vi "Registry Set.vi"() -> ()   [LabVIEW 2013]
uses:
  <vilib>/Rock Robotics/WPI/Joystick/WPI_JoystickDeviceEnum.ctl
  <vilib>/Rock Robotics/SystemInterfaces/AI/FPGA_AIChannel.ctl
  <vilib>/Rock Robotics/SystemInterfaces/DIO/FPGA_DIOPWMChannel.ctl
  <vilib>/Rock Robotics/SystemInterfaces/Typedef/FPGA_TypedefAnalogModule.ctl
  <vilib>/Rock Robotics/SystemInterfaces/Typedef/FPGA_TypedefDigitalModule.ctl
  <vilib>/Rock Robotics/SystemInterfaces/DIO/FPGA_DIORelayChannel.ctl
  <vilib>/Rock Robotics/SystemInterfaces/DIO/FPGA_DIOChannel.ctl
  <vilib>/Rock Robotics/WPI/Solenoid/WPI_SolenoidChannel.ctl
  <vilib>/Rock Robotics/SystemInterfaces/Typedef/FPGA_TypedefSolenoidModule.ctl
  <vilib>/Rock Robotics/SystemInterfaces/Typedef/FPGA_TypedefAnalogModuleForGyro.ctl
  <vilib>/Rock Robotics/SystemInterfaces/AI/FPGA_AIGyroChannel.ctl
  <vilib>/Rock Robotics/WPI/MotorControl/WPI_MotorControlOpen Talon.vi
  <vilib>/Rock Robotics/WPI/MotorControl/WPI_MotorControlOpen Jaguar.vi
  <vilib>/Rock Robotics/WPI/Solenoid/WPI_SolenoidOpenSingle.vi
  <vilib>/Rock Robotics/WPI/Counter/WPI_CounterDigitalInputToDigitalSource.vi
  Global Refnums.vi
  <vilib>/Rock Robotics/WPI/Compressor/WPI_CompressorGetSetRefNum.vi
panel:
  out "error out":errorcluster
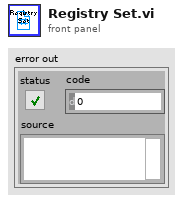
[diagram p1: front panel]
types:
  T1 = typedef "FPGA_AIGyroChannel.ctl" = enum8{"AI 1", "AI 2", "Invalid"}
  T2 = typedef "FPGA_TypedefAnalogModuleForGyro.ctl" = enum16{"Analog Module 1"}
  T3 = typedef "FPGA_DIOChannel.ctl" = enum8{"DIO 1", "DIO 2", "DIO 3", "DIO 4", "DIO 5", "DIO 6", "DIO 7", "DIO 8", "DIO 9", "DIO 10", "DIO 11", "DIO 12", "DIO 13", "DIO 14", "Invalid"}
  T4 = typedef "FPGA_TypedefDigitalModule.ctl" = enum16{"Digital Module 1", "Digital Module 2"}
  T5 = typedef "WPI_SolenoidChannel.ctl" = enum8{"Solenoid 1", "Solenoid 2", "Solenoid 3", "Solenoid 4", "Solenoid 5", "Solenoid 6", "Solenoid 7", "Solenoid 8", "Invalid"}
  T6 = typedef "FPGA_TypedefSolenoidModule.ctl" = enum16{"Solenoid Module 1", "Solenoid Module 2"}
  T7 = typedef "FPGA_DIORelayChannel.ctl" = enum8{"Relay 1", "Relay 2", "Relay 3", "Relay 4", "Relay 5", "Relay 6", "Relay 7", "Relay 8", "Invalid"}
  T8 = typedef "FPGA_DIOPWMChannel.ctl" = enum8{"PWM 1", "PWM 2", "PWM 3", "PWM 4", "PWM 5", "PWM 6", "PWM 7", "PWM 8", "PWM 9", "PWM 10", "Invalid"}
  T9 = typedef "WPI_JoystickDeviceEnum.ctl" = enum16{"USB 1", "USB 2", "USB 3", "USB 4", "Kinect 1", "Kinect 2"}
  T10 = typedef "FPGA_AIChannel.ctl" = enum8{"AI 1", "AI 2", "AI 3", "AI 4", "AI 5", "AI 6", "AI 7", "AI 8", "Invalid"}
  T11 = typedef "FPGA_TypedefAnalogModule.ctl" = enum16{"Analog Module 1", "Analog Module 2"}
  T12 = typedef "WPI_GyroDevRef.ctl" = cluster{"DevStatus":errorcluster, "Analog Module":T11, "Analog Channel":T10, "Offset":dbl, "Gain (VoltsPerDegree/Second)":dbl}
  T13 = typedef "WPI_JoystickDevRef.ctl" = cluster{"Device":T9}
  T14 = typedef "WPI_AnalogChannelDevRef.ctl" = cluster{"DevStatus":errorcluster, "Analog Module":T11, "Analog Channel":T10}
  T15 = typedef "WPI_DigitalInputDevRef.ctl" = cluster{"DevStatus":errorcluster, "DIO Channel":T3, "Digital Module":T4}
  T16 = typedef "WPI_MotorControlDeviceRef.ctl" = cluster{"DeviceStatus":errorcluster, "Type":enum16{"PWM", "CAN"}, "PWM":cluster{"Digital Module":T4, "PWM Channel":T8, "DeadBand":T17}, "CAN":cluster{"Device Number":u8, "Control Mode":T18, "Semaphore":T19, "Max Vout":dbl}, "Invert":bool, "TransformRef":T20, "InvTransformRef":T20}
  T17 = typedef "WPI_PWMDeadband.ctl" = cluster{"Name":string, "maxPositivePwm":i32, "minPositivePwm":i32, "centerPwm":i32, "maxNegativePwm":i32, "minNegativePwm":i32, "angularRange":u16}
  T18 = typedef "WPI_CANJaguar_ControlMode.ctl" = enum8{"Percent VBus", "Current", "Speed", "Position", "Voltage"}
  T19 = typedef "Semaphore RefNum" = refnum<k1>
  T20 = typedef "WPI_PWMTransform_ConPane.ctl" = refnum<vi>
  T21 = typedef "FPGA_CounterEncoderSourceConvertionLVSourceType.ctl" = cluster{"DevStatus":errorcluster, "AnalogTriggerMode?":bool, "DigitalMode":cluster{"Digital Module":T4, "DIO Channel":T22}, "AnalogTriggerMode":cluster{"AnalogTriggerIndex":T23, "OutputType":T24}}
  T22 = typedef "FPGA_DIODigitalSourceChannel.ctl" = enum8{"DIO 1", "DIO 2", "DIO 3", "DIO 4", "DIO 5", "DIO 6", "DIO 7", "DIO 8", "DIO 9", "DIO 10", "DIO 11", "DIO 12", "DIO 13", "DIO 14", "Disabled"}
  T23 = typedef "FPGA_AnalogTriggerIndex.ctl" = enum8{"Trig 0", "Trig 1", "Trig 2", "Trig 3", "Trig 4", "Trig 5", "Trig 6", "Trig 7", "Invalid"}
  T24 = typedef "FPGA_AnalogTriggerOutType.ctl" = enum16{"InWindow", "TriggerState", "Rising", "Falling"}
  T25 = typedef "WPI_EncoderDevRef.ctl" = cluster{"DevStatus":errorcluster, "EncoderIndex":T26, "CounterIndex":T27, "DistancePerCount":dbl, "Decoding Type":T28}
  T26 = typedef "FPGA_EncoderIdx.ctl" = enum8{"Enc 0", "Enc 1", "Enc 2", "Enc 3", "Invalid"}
  T27 = typedef "FPGA_CounterCtrSystemIndex.ctl" = enum8{"Ctr 0", "Ctr 1", "Ctr 2", "Ctr 3", "Ctr 4", "Ctr 5", "Ctr 6", "Ctr 7", "Invalid"}
  T28 = typedef "WPI_EncoderType.ctl" = enum16{"1x", "2x", "4x"}
  T29 = typedef "WPI_CompressorDevRef.ctl" = cluster{"DevStatus":errorcluster, "DigitalInputDevRef":T15, "RelayDevRef":T30}
  T30 = typedef "WPI_RelayDevRef.ctl" = cluster{"DevStatus":errorcluster, "Relay Channel":T7, "Digital Module":T4, "Relay Direction":T31}
  T31 = typedef "WPI_RelayDirection.ctl" = enum16{"Both directions", "Forward only", "Reverse only"}
  T32 = typedef "WPI_SolenoidDevRef.ctl" = cluster{"DevStatus":errorcluster, "Solenoid Module":T6, "Forward Solenoid Channel":T5, "Reverse Solenoid Channel":T5}
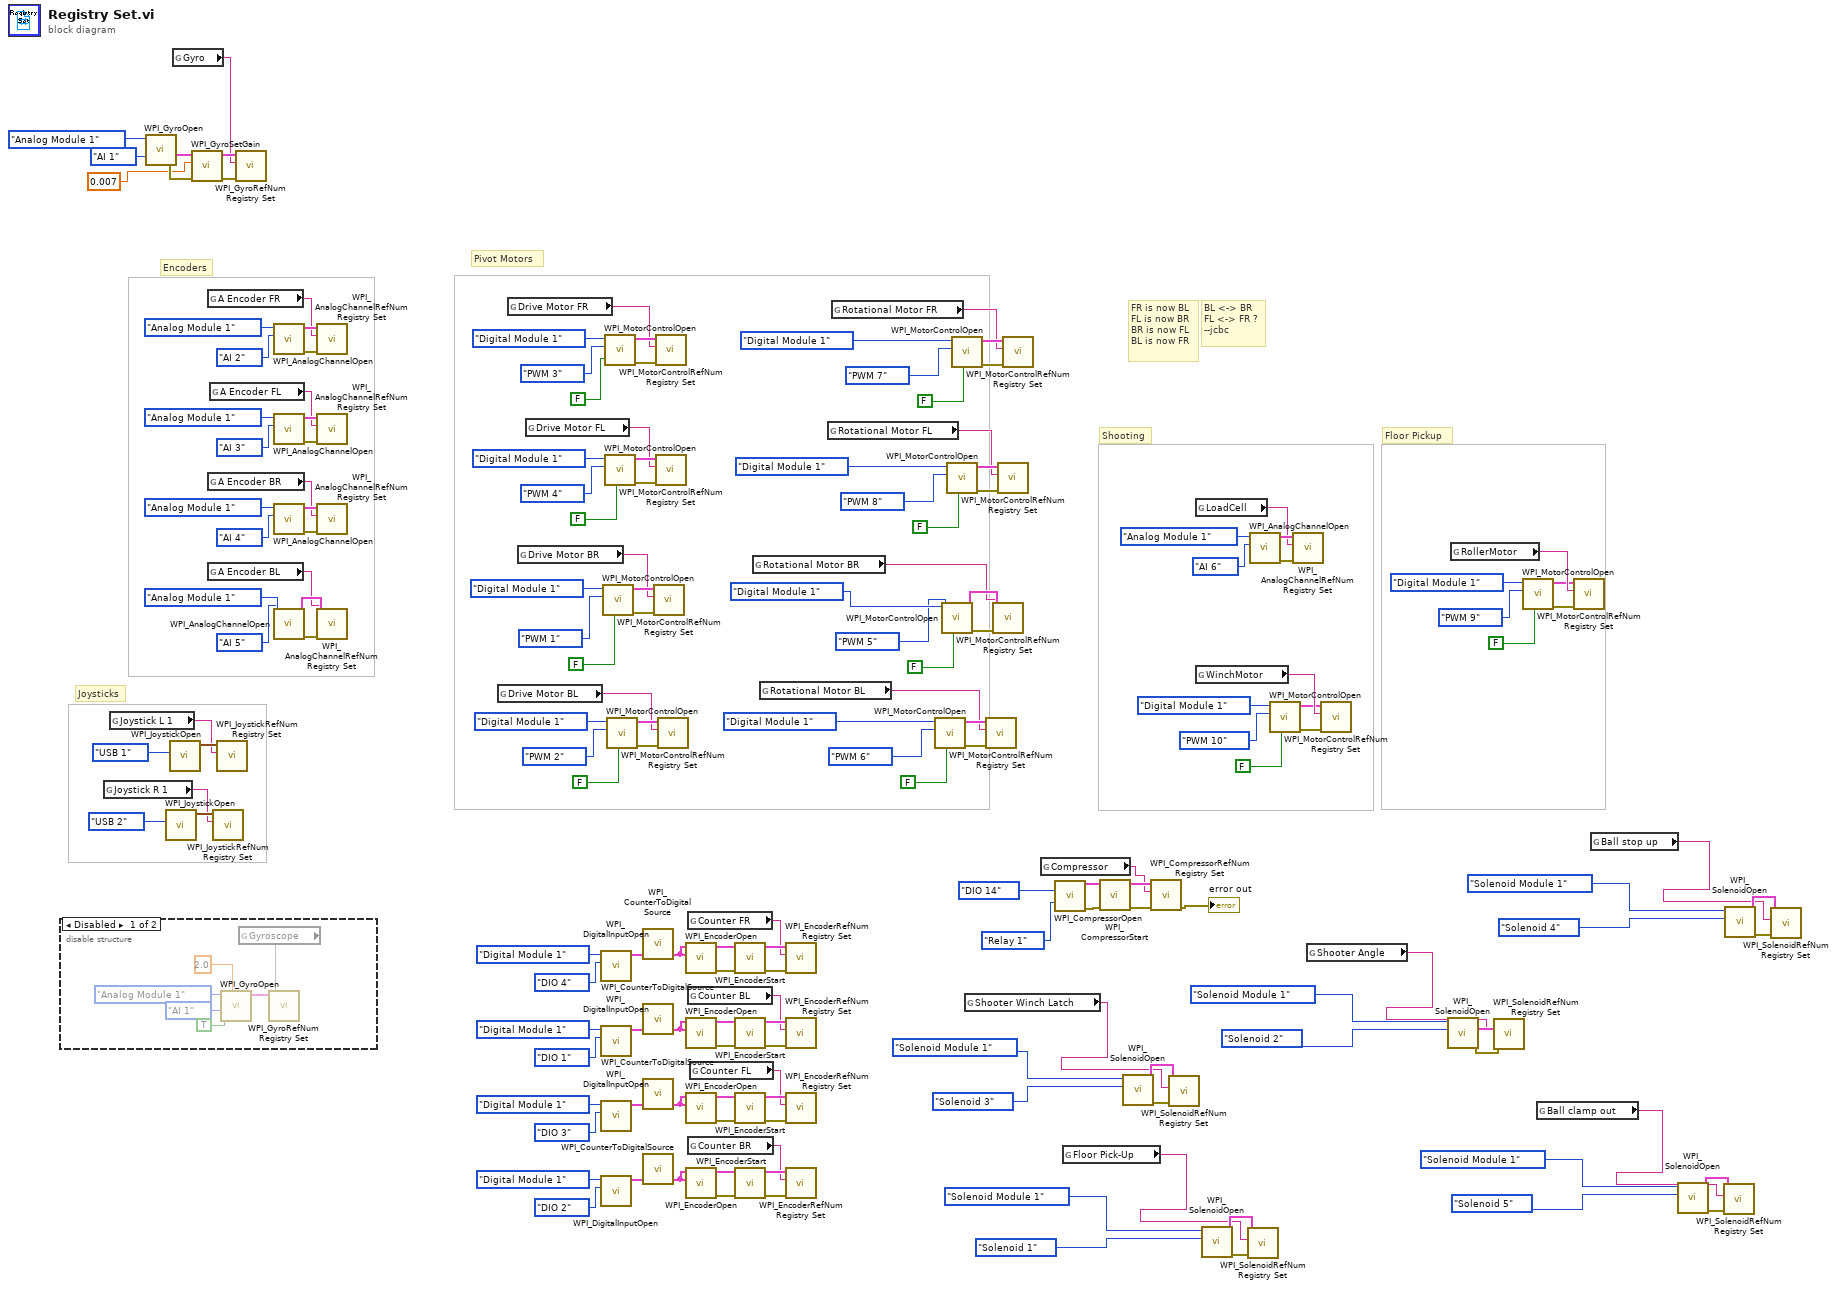
[diagram p0: block diagram]
diagram:
  # "Floor Pickup"
  # "Shooting"
  # "BL <-> BR\nFL <-> FR ?\n--jcbc"
  # "FR is now BL\nFL is now BR\nBR is now FL\nBL is now FR"
  # "Pivot Motors"
  # "Encoders"
  # "Joysticks"
  n1 = disable-structure shown="Disabled" {
    frame Disabled {
      n2 = call <vilib>:"WPI_GyroOpen.vi"("Calibration Time (s)"=2.0, "Calibrate On Open"=TRUE, "Analog Channel"=FPGA_AIGyroChannel."AI 1", "Analog Module (Module 1)"=FPGA_TypedefAnalogModuleForGyro."Analog Module 1") -> ("GyroDevRef"=w170:T12)  [unwired: 5 in, 2 out]
      n3 = global read "Global Refnums.vi" "Gyroscope"() -> (w169)
      n4 = call <vilib>:"WPI_GyroRefNum Registry Set.vi"("refnum name"=w169, "GyroDevRef"=w170) -> ()  [unwired: 8 in, 2 out]
    }
    frame Enabled {
    }
  }
  n5 = global read "Global Refnums.vi" "Joystick R 1"() -> (w166:string)
  n6 = global read "Global Refnums.vi" "Joystick L 1"() -> (w84:string)
  n7 = call <vilib>:"WPI_GyroOpen.vi"("Analog Channel"=FPGA_AIGyroChannel."AI 1", "Analog Module (Module 1)"=FPGA_TypedefAnalogModuleForGyro."Analog Module 1") -> ("error out"=w8:errorcluster, "GyroDevRef"=w7:T12)  [unwired: 7 in, 1 out]
  n8 = call <vilib>:"WPI_JoystickOpen.vi"("JoystickDevice"=WPI_JoystickDeviceEnum."USB 2") -> ("JoystickDevRef"=w167:T13)  [unwired: 10 in]
  n9 = call <vilib>:"WPI_JoystickOpen.vi"("JoystickDevice"=WPI_JoystickDeviceEnum."USB 1") -> ("JoystickDevRef"=w85:T13)  [unwired: 10 in]
  n10 = global read "Global Refnums.vi" "Gyro"() -> (w1:string)
  n11 = call <vilib>:"WPI_GyroSetGain.vi"("error in (no error)"=w8, "Gain (VoltsPerDegree/Second)"=0.007, "GyroDevRef"=w7) -> ("error out"=w6:errorcluster, "GyroDevRef"=w5:T12)  [unwired: 7 in]
  n12 = global read "Global Refnums.vi" "A Encoder FR"() -> (w161:string)
  n13 = global read "Global Refnums.vi" "A Encoder BR"() -> (w147:string)
  n14 = global read "Global Refnums.vi" "A Encoder BL"() -> (w146:string)
  n15 = global read "Global Refnums.vi" "A Encoder FL"() -> (w148:string)
  n16 = call <vilib>:"WPI_JoystickRefNum Registry Set.vi"("refnum name"=w166, "JoystickDevRef"=w167) -> ()  [unwired: 8 in, 2 out]
  n17 = call <vilib>:"WPI_JoystickRefNum Registry Set.vi"("refnum name"=w84, "JoystickDevRef"=w85) -> ()  [unwired: 8 in, 2 out]
  n18 = call <vilib>:"WPI_GyroRefNum Registry Set.vi"("error in (no error)"=w6, "refnum name"=w1, "GyroDevRef"=w5) -> ()  [unwired: 7 in, 2 out]
  n19 = call <vilib>:"WPI_AnalogChannelOpen.vi"("Analog Channel"=FPGA_AIChannel."AI 2", "Analog Module (Module 1)"=FPGA_TypedefAnalogModule."Analog Module 1") -> ("error out"=w164:errorcluster, "AIDeviceRef"=w165:T14)  [unwired: 8 in]
  n20 = call <vilib>:"WPI_AnalogChannelOpen.vi"("Analog Channel"=FPGA_AIChannel."AI 3", "Analog Module (Module 1)"=FPGA_TypedefAnalogModule."Analog Module 1") -> ("error out"=w159:errorcluster, "AIDeviceRef"=w160:T14)  [unwired: 8 in]
  n21 = call <vilib>:"WPI_AnalogChannelOpen.vi"("Analog Channel"=FPGA_AIChannel."AI 4", "Analog Module (Module 1)"=FPGA_TypedefAnalogModule."Analog Module 1") -> ("error out"=w155:errorcluster, "AIDeviceRef"=w156:T14)  [unwired: 8 in]
  n22 = call <vilib>:"WPI_AnalogChannelOpen.vi"("Analog Channel"=FPGA_AIChannel."AI 5", "Analog Module (Module 1)"=FPGA_TypedefAnalogModule."Analog Module 1") -> ("error out"=w151:errorcluster, "AIDeviceRef"=w152:T14)  [unwired: 8 in]
  n23 = call <vilib>:"WPI_AnalogChannelRefNum Registry Set.vi"("error in (no error)"=w164, "refnum name"=w161, "AIDeviceRef"=w165) -> ()  [unwired: 7 in, 2 out]
  n24 = call <vilib>:"WPI_AnalogChannelRefNum Registry Set.vi"("error in (no error)"=w159, "refnum name"=w148, "AIDeviceRef"=w160) -> ()  [unwired: 7 in, 2 out]
  n25 = call <vilib>:"WPI_AnalogChannelRefNum Registry Set.vi"("error in (no error)"=w155, "refnum name"=w147, "AIDeviceRef"=w156) -> ()  [unwired: 7 in, 2 out]
  n26 = call <vilib>:"WPI_AnalogChannelRefNum Registry Set.vi"("error in (no error)"=w151, "refnum name"=w146, "AIDeviceRef"=w152) -> ()  [unwired: 7 in, 2 out]
  n27 = global read "Global Refnums.vi" "Drive Motor BL"() -> (w123:string)
  n28 = global read "Global Refnums.vi" "Drive Motor FR"() -> (w141:string)
  n29 = global read "Global Refnums.vi" "Drive Motor BR"() -> (w122:string)
  n30 = global read "Global Refnums.vi" "Drive Motor FL"() -> (w129:string)
  n31 = call <vilib>:"WPI_DigitalInputOpen.vi"("DIO Channel"=FPGA_DIOChannel."DIO 4", "Digital Module (Module 1)"=FPGA_TypedefDigitalModule."Digital Module 1") -> ("DigitalInputDevRef"=w44:T15)  [unwired: 8 in, 1 out]
  n32 = call <vilib>:"WPI_DigitalInputOpen.vi"("DIO Channel"=FPGA_DIOChannel."DIO 1", "Digital Module (Module 1)"=FPGA_TypedefDigitalModule."Digital Module 1") -> ("DigitalInputDevRef"=w31:T15)  [unwired: 8 in, 1 out]
  n33 = call <vilib>:"WPI_DigitalInputOpen.vi"("DIO Channel"=FPGA_DIOChannel."DIO 3", "Digital Module (Module 1)"=FPGA_TypedefDigitalModule."Digital Module 1") -> ("DigitalInputDevRef"=w23:T15)  [unwired: 8 in, 1 out]
  n34 = call <vilib>:"WPI_DigitalInputOpen.vi"("DIO Channel"=FPGA_DIOChannel."DIO 2", "Digital Module (Module 1)"=FPGA_TypedefDigitalModule."Digital Module 1") -> ("DigitalInputDevRef"=w15:T15)  [unwired: 8 in, 1 out]
  n35 = call-poly <vilib>:"WPI_MotorControlOpen.vi"("Invert"=FALSE, "PWM Channel"=FPGA_DIOPWMChannel."PWM 1", "Digital Module (Module 1)"=FPGA_TypedefDigitalModule."Digital Module 1") -> ("error out"=w131:errorcluster, "MotorControlDeviceRef"=w132:T16)  [unwired: 7 in]
  n36 = call-poly <vilib>:"WPI_MotorControlOpen.vi"("Invert"=FALSE, "PWM Channel"=FPGA_DIOPWMChannel."PWM 3", "Digital Module (Module 1)"=FPGA_TypedefDigitalModule."Digital Module 1") -> ("error out"=w142:errorcluster, "MotorControlDeviceRef"=w143:T16)  [unwired: 7 in]
  n37 = call-poly <vilib>:"WPI_MotorControlOpen.vi"("Invert"=FALSE, "PWM Channel"=FPGA_DIOPWMChannel."PWM 4", "Digital Module (Module 1)"=FPGA_TypedefDigitalModule."Digital Module 1") -> ("error out"=w136:errorcluster, "MotorControlDeviceRef"=w137:T16)  [unwired: 7 in]
  n38 = call-poly <vilib>:"WPI_MotorControlOpen.vi"("Invert"=FALSE, "PWM Channel"=FPGA_DIOPWMChannel."PWM 2", "Digital Module (Module 1)"=FPGA_TypedefDigitalModule."Digital Module 1") -> ("error out"=w125:errorcluster, "MotorControlDeviceRef"=w126:T16)  [unwired: 7 in]
  n39 = call-poly <vilib>:"WPI_CounterToDigitalSource.vi"("DigitalInputDevRef"=w44) -> ("Digital Source"=w43:T21)  [unwired: 6 in]
  n40 = call-poly <vilib>:"WPI_CounterToDigitalSource.vi"("DigitalInputDevRef"=w31) -> ("Digital Source"=w32:T21)  [unwired: 6 in]
  n41 = call-poly <vilib>:"WPI_CounterToDigitalSource.vi"("DigitalInputDevRef"=w23) -> ("Digital Source"=w24:T21)  [unwired: 6 in]
  n42 = call-poly <vilib>:"WPI_CounterToDigitalSource.vi"("DigitalInputDevRef"=w15) -> ("Digital Source"=w20:T21)  [unwired: 6 in]
  n43 = call <vilib>:"WPI_MotorControlRefNum Registry Set.vi"("error in (no error)"=w131, "refnum name"=w122, "MotorControlDevRef"=w132) -> ()  [unwired: 7 in, 2 out]
  n44 = call <vilib>:"WPI_MotorControlRefNum Registry Set.vi"("error in (no error)"=w142, "refnum name"=w141, "MotorControlDevRef"=w143) -> ()  [unwired: 7 in, 2 out]
  n45 = call <vilib>:"WPI_MotorControlRefNum Registry Set.vi"("error in (no error)"=w136, "refnum name"=w129, "MotorControlDevRef"=w137) -> ()  [unwired: 7 in, 2 out]
  n46 = call <vilib>:"WPI_MotorControlRefNum Registry Set.vi"("error in (no error)"=w125, "refnum name"=w123, "MotorControlDevRef"=w126) -> ()  [unwired: 7 in, 2 out]
  n47 = call <vilib>:"WPI_EncoderOpen.vi"("BSource"=w43, "ASource"=w43) -> ("error out"=w41:errorcluster, "EncoderDevRef"=w42:T25)  [unwired: 8 in]
  n48 = call <vilib>:"WPI_EncoderOpen.vi"("BSource"=w32, "ASource"=w32) -> ("error out"=w34:errorcluster, "EncoderDevRef"=w33:T25)  [unwired: 8 in]
  n49 = call <vilib>:"WPI_EncoderOpen.vi"("BSource"=w24, "ASource"=w24) -> ("error out"=w26:errorcluster, "EncoderDevRef"=w25:T25)  [unwired: 8 in]
  n50 = call <vilib>:"WPI_EncoderOpen.vi"("BSource"=w20, "ASource"=w20) -> ("error out"=w18:errorcluster, "EncoderDevRef"=w19:T25)  [unwired: 8 in]
  n51 = global read "Global Refnums.vi" "Counter FR"() -> (w12:string)
  n52 = global read "Global Refnums.vi" "Counter BL"() -> (w11:string)
  n53 = global read "Global Refnums.vi" "Counter BR"() -> (w9:string)
  n54 = global read "Global Refnums.vi" "Counter FL"() -> (w10:string)
  n55 = call <vilib>:"WPI_EncoderStart.vi"("error in (no error)"=w41, "EncoderDevRef"=w42) -> ("error out"=w39:errorcluster, "EncoderDevRef"=w40:T25)  [unwired: 8 in]
  n56 = call <vilib>:"WPI_EncoderStart.vi"("error in (no error)"=w34, "EncoderDevRef"=w33) -> ("error out"=w36:errorcluster, "EncoderDevRef"=w35:T25)  [unwired: 8 in]
  n57 = call <vilib>:"WPI_EncoderStart.vi"("error in (no error)"=w26, "EncoderDevRef"=w25) -> ("error out"=w28:errorcluster, "EncoderDevRef"=w27:T25)  [unwired: 8 in]
  n58 = call <vilib>:"WPI_EncoderStart.vi"("error in (no error)"=w18, "EncoderDevRef"=w19) -> ("error out"=w16:errorcluster, "EncoderDevRef"=w17:T25)  [unwired: 8 in]
  n59 = global read "Global Refnums.vi" "Rotational Motor BR"() -> (w101:string)
  n60 = global read "Global Refnums.vi" "Rotational Motor BL"() -> (w98:string)
  n61 = call <vilib>:"WPI_EncoderRefNum Registry Set.vi"("error in (no error)"=w39, "refnum name"=w12, "EncoderDevRef"=w40) -> ()  [unwired: 7 in, 2 out]
  n62 = call <vilib>:"WPI_EncoderRefNum Registry Set.vi"("error in (no error)"=w36, "refnum name"=w11, "EncoderDevRef"=w35) -> ()  [unwired: 7 in, 2 out]
  n63 = call <vilib>:"WPI_EncoderRefNum Registry Set.vi"("error in (no error)"=w28, "refnum name"=w10, "EncoderDevRef"=w27) -> ()  [unwired: 7 in, 2 out]
  n64 = call <vilib>:"WPI_EncoderRefNum Registry Set.vi"("error in (no error)"=w16, "refnum name"=w9, "EncoderDevRef"=w17) -> ()  [unwired: 7 in, 2 out]
  n65 = global read "Global Refnums.vi" "Rotational Motor FL"() -> (w100:string)
  n66 = global read "Global Refnums.vi" "Rotational Motor FR"() -> (w99:string)
  n67 = call-poly <vilib>:"WPI_MotorControlOpen.vi"("Invert"=FALSE, "PWM Channel"=FPGA_DIOPWMChannel."PWM 6", "Digital Module (Module 1)"=FPGA_TypedefDigitalModule."Digital Module 1") -> ("error out"=w103:errorcluster, "MotorControlDeviceRef"=w104:T16)  [unwired: 7 in]
  n68 = call-poly <vilib>:"WPI_MotorControlOpen.vi"("Invert"=FALSE, "PWM Channel"=FPGA_DIOPWMChannel."PWM 5", "Digital Module (Module 1)"=FPGA_TypedefDigitalModule."Digital Module 1") -> ("error out"=w108:errorcluster, "MotorControlDeviceRef"=w109:T16)  [unwired: 7 in]
  n69 = call-poly <vilib>:"WPI_MotorControlOpen.vi"("Invert"=FALSE, "PWM Channel"=FPGA_DIOPWMChannel."PWM 8", "Digital Module (Module 1)"=FPGA_TypedefDigitalModule."Digital Module 1") -> ("error out"=w113:errorcluster, "MotorControlDeviceRef"=w114:T16)  [unwired: 7 in]
  n70 = call-poly <vilib>:"WPI_MotorControlOpen.vi"("Invert"=FALSE, "PWM Channel"=FPGA_DIOPWMChannel."PWM 7", "Digital Module (Module 1)"=FPGA_TypedefDigitalModule."Digital Module 1") -> ("error out"=w118:errorcluster, "MotorControlDeviceRef"=w119:T16)  [unwired: 7 in]
  n71 = global read "Global Refnums.vi" "Shooter Winch Latch"() -> (w67:string)
  n72 = call <vilib>:"WPI_MotorControlRefNum Registry Set.vi"("error in (no error)"=w103, "refnum name"=w98, "MotorControlDevRef"=w104) -> ()  [unwired: 7 in, 2 out]
  n73 = call <vilib>:"WPI_MotorControlRefNum Registry Set.vi"("error in (no error)"=w108, "refnum name"=w101, "MotorControlDevRef"=w109) -> ()  [unwired: 7 in, 2 out]
  n74 = call <vilib>:"WPI_MotorControlRefNum Registry Set.vi"("error in (no error)"=w113, "refnum name"=w100, "MotorControlDevRef"=w114) -> ()  [unwired: 7 in, 2 out]
  n75 = call <vilib>:"WPI_MotorControlRefNum Registry Set.vi"("error in (no error)"=w118, "refnum name"=w99, "MotorControlDevRef"=w119) -> ()  [unwired: 7 in, 2 out]
  n76 = global read "Global Refnums.vi" "Compressor"() -> (w70:string)
  n77 = call <vilib>:"WPI_CompressorOpen.vi"("Pressure Switch DIO Channel"=FPGA_DIOChannel."DIO 14", "Relay Channel"=FPGA_DIORelayChannel."Relay 1") -> ("CompressorDevRef"=w75:T29, "error out"=w74:errorcluster)  [unwired: 12 in]
  n78 = global read "Global Refnums.vi" "Floor Pick-Up"() -> (w57:string)
  n79 = call <vilib>:"WPI_CompressorStart.vi"("error in (no error)"=w74, "CompressorDevRef"=w75) -> ("error out"=w76:errorcluster, "CompressorDevRef"=w77:T29)  [unwired: 8 in]
  n80 = call-poly <vilib>:"WPI_SolenoidOpen.vi"("Solenoid Channel"=WPI_SolenoidChannel."Solenoid 3", "Solenoid Module (Module 1)"=FPGA_TypedefSolenoidModule."Solenoid Module 1") -> ("error out"=w69:errorcluster, "SolenoidDevRef"=w68:T32)  [unwired: 8 in]
  n81 = call <vilib>:"WPI_CompressorRefNum Registry Set.vi"("error in (no error)"=w76, "refnum name"=w70, "CompressorDevRef"=w77) -> ("error out"=→"error out":errorcluster)  [unwired: 7 in, 1 out]
  n82 = call <vilib>:"WPI_SolenoidRefNum Registry Set.vi"("error in (no error)"=w69, "refnum name"=w67, "SolenoidDevRef"=w68) -> ()  [unwired: 7 in, 2 out]
  n83 = global read "Global Refnums.vi" "LoadCell"() -> (w93:string)
  n84 = global read "Global Refnums.vi" "WinchMotor"() -> (w92:string)
  n85 = call-poly <vilib>:"WPI_SolenoidOpen.vi"("Solenoid Channel"=WPI_SolenoidChannel."Solenoid 1", "Solenoid Module (Module 1)"=FPGA_TypedefSolenoidModule."Solenoid Module 1") -> ("error out"=w59:errorcluster, "SolenoidDevRef"=w58:T32)  [unwired: 8 in]
  n86 = call <vilib>:"WPI_SolenoidRefNum Registry Set.vi"("error in (no error)"=w59, "refnum name"=w57, "SolenoidDevRef"=w58) -> ()  [unwired: 7 in, 2 out]
  n87 = call <vilib>:"WPI_AnalogChannelOpen.vi"("Analog Channel"=FPGA_AIChannel."AI 6", "Analog Module (Module 1)"=FPGA_TypedefAnalogModule."Analog Module 1") -> ("error out"=w96:errorcluster, "AIDeviceRef"=w97:T14)  [unwired: 8 in]
  n88 = call-poly <vilib>:"WPI_MotorControlOpen.vi"("Invert"=FALSE, "PWM Channel"=FPGA_DIOPWMChannel."PWM 10", "Digital Module (Module 1)"=FPGA_TypedefDigitalModule."Digital Module 1") -> ("error out"=w90:errorcluster, "MotorControlDeviceRef"=w89:T16)  [unwired: 7 in]
  n89 = call <vilib>:"WPI_AnalogChannelRefNum Registry Set.vi"("error in (no error)"=w96, "refnum name"=w93, "AIDeviceRef"=w97) -> ()  [unwired: 7 in, 2 out]
  n90 = global read "Global Refnums.vi" "Shooter Angle"() -> (w62:string)
  n91 = call <vilib>:"WPI_MotorControlRefNum Registry Set.vi"("error in (no error)"=w90, "refnum name"=w92, "MotorControlDevRef"=w89) -> ()  [unwired: 7 in, 2 out]
  n92 = call-poly <vilib>:"WPI_SolenoidOpen.vi"("Solenoid Channel"=WPI_SolenoidChannel."Solenoid 2", "Solenoid Module (Module 1)"=FPGA_TypedefSolenoidModule."Solenoid Module 1") -> ("error out"=w64:errorcluster, "SolenoidDevRef"=w63:T32)  [unwired: 8 in]
  n93 = global read "Global Refnums.vi" "RollerMotor"() -> (w83:string)
  n94 = call <vilib>:"WPI_SolenoidRefNum Registry Set.vi"("error in (no error)"=w64, "refnum name"=w62, "SolenoidDevRef"=w63) -> ()  [unwired: 7 in, 2 out]
  n95 = call-poly <vilib>:"WPI_MotorControlOpen.vi"("Invert"=FALSE, "PWM Channel"=FPGA_DIOPWMChannel."PWM 9", "Digital Module (Module 1)"=FPGA_TypedefDigitalModule."Digital Module 1") -> ("error out"=w81:errorcluster, "MotorControlDeviceRef"=w80:T16)  [unwired: 7 in]
  n96 = global read "Global Refnums.vi" "Ball clamp out"() -> (w52:string)
  n97 = call <vilib>:"WPI_MotorControlRefNum Registry Set.vi"("error in (no error)"=w81, "refnum name"=w83, "MotorControlDevRef"=w80) -> ()  [unwired: 7 in, 2 out]
  n98 = global read "Global Refnums.vi" "Ball stop up"() -> (w47:string)
  n99 = call-poly <vilib>:"WPI_SolenoidOpen.vi"("Solenoid Channel"=WPI_SolenoidChannel."Solenoid 5", "Solenoid Module (Module 1)"=FPGA_TypedefSolenoidModule."Solenoid Module 1") -> ("error out"=w54:errorcluster, "SolenoidDevRef"=w53:T32)  [unwired: 8 in]
  n100 = call <vilib>:"WPI_SolenoidRefNum Registry Set.vi"("error in (no error)"=w54, "refnum name"=w52, "SolenoidDevRef"=w53) -> ()  [unwired: 7 in, 2 out]
  n101 = call-poly <vilib>:"WPI_SolenoidOpen.vi"("Solenoid Channel"=WPI_SolenoidChannel."Solenoid 4", "Solenoid Module (Module 1)"=FPGA_TypedefSolenoidModule."Solenoid Module 1") -> ("error out"=w49:errorcluster, "SolenoidDevRef"=w48:T32)  [unwired: 8 in]
  n102 = call <vilib>:"WPI_SolenoidRefNum Registry Set.vi"("error in (no error)"=w49, "refnum name"=w47, "SolenoidDevRef"=w48) -> ()  [unwired: 7 in, 2 out]
